vi "WriteCommand.vi"(7 "PWM":u8=24, 8 "error in":errorcluster, 9 "Com_Escribir":T1=enum."GET REF", 10 "VisaRef":refnum<vi>, 11 "Array_u8":u8[](array[numeric])) -> (0 "error out":errorcluster, 2 "VISA resource name 2":refnum<visa-resource-name>)   [LabVIEW 2026]
uses:
  Control/Ctrl_EscrituraComandos.ctl
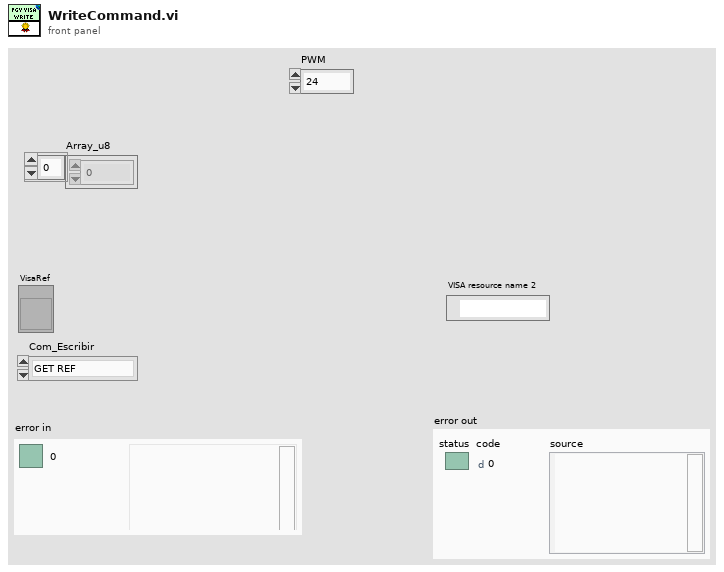
[diagram p1: front panel]
types:
  T1 = typedef "Ctrl_EscrituraComandos.ctl" = enum16{"EMERGENCY STOP", "GET REF", "SEND ROUTINE", "MOVE MANUAL", "SEND ESP32", "SET REF"}
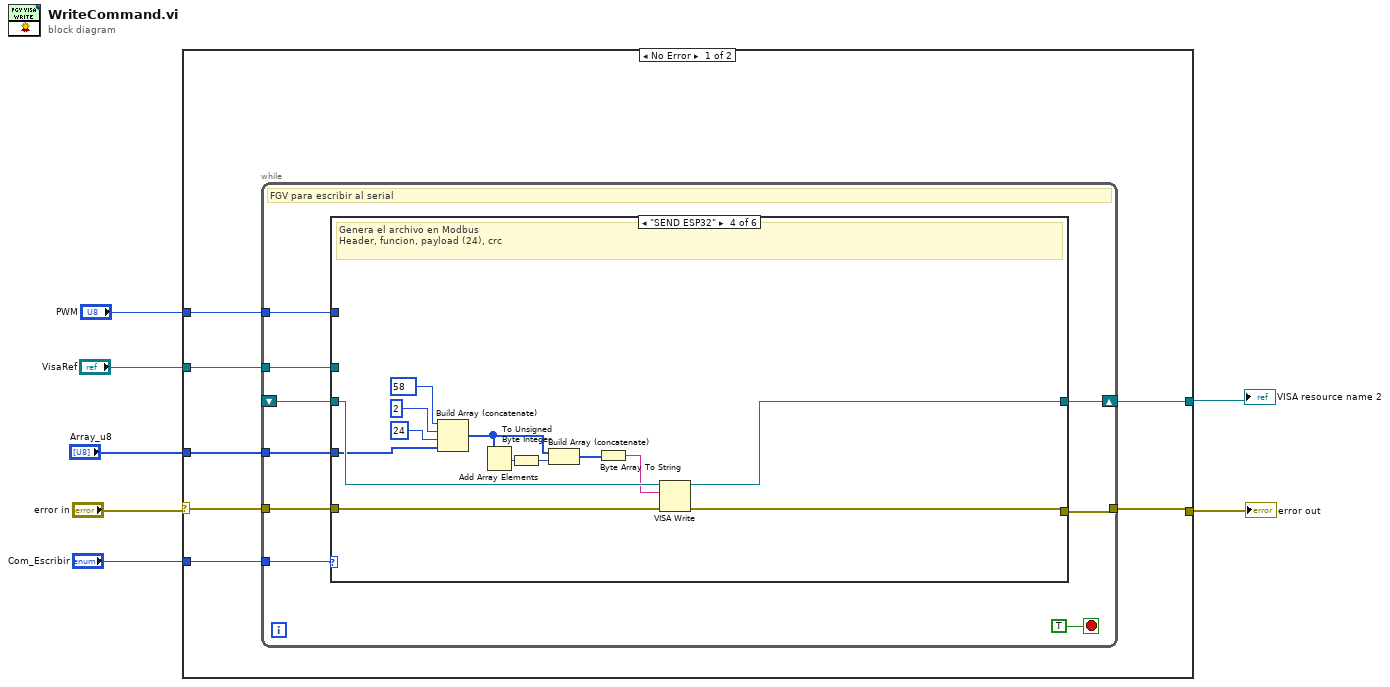
[diagram p0: block diagram]
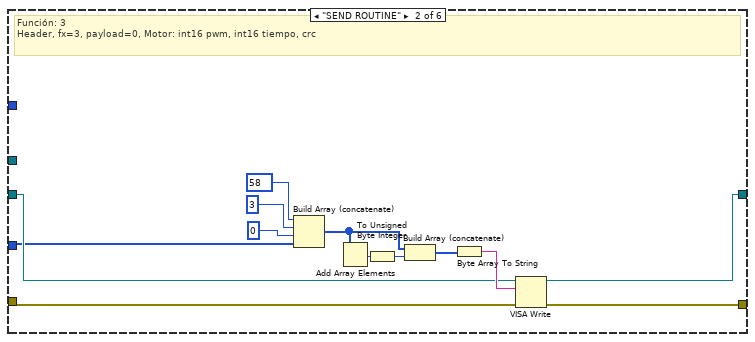
[diagram p3: hidden frame]
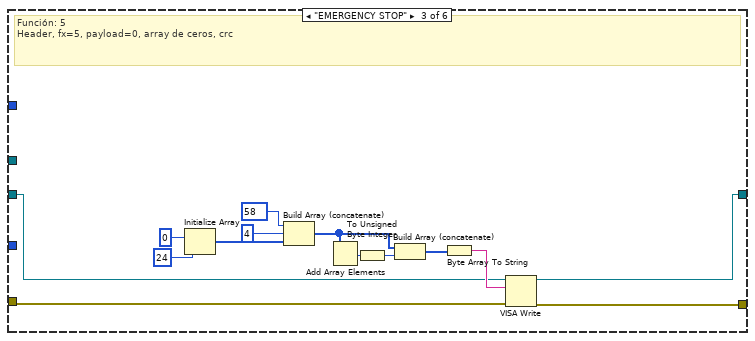
[diagram p4: hidden frame]
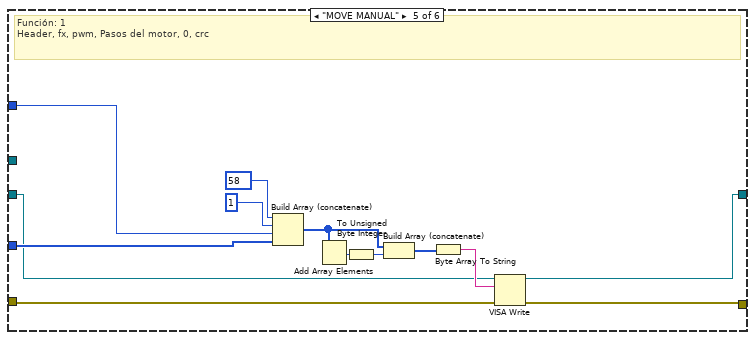
[diagram p5: hidden frame]
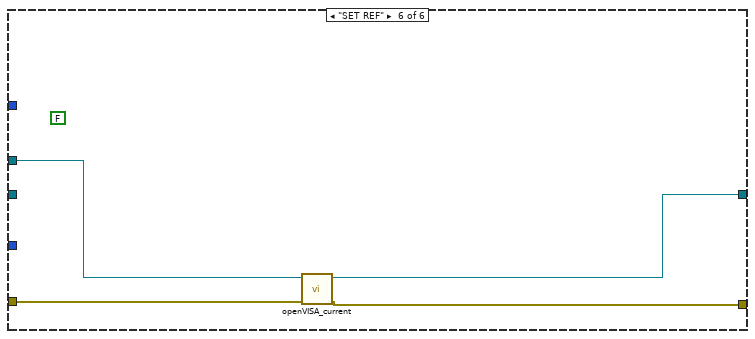
[diagram p6: hidden frame]
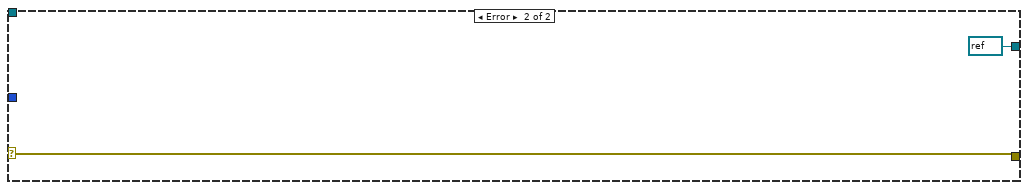
[diagram p7: hidden frame]
diagram:
  n1 = case shown="No Error" "error in" {
    selector: "error in" -> [w14 w84]
    tunnel: [w13 w84] -> w6
    tunnel: [w11 refnum<visa-resource-name> refnum ("VISA Refnum out")] -> w5
    tunnel: "Com_Escribir" -> [w12 _]
    tunnel: "Array_u8" -> [w10 _]
    tunnel: "VisaRef" -> [w9 _]
    tunnel: "PWM" -> [w8 _]
    frame No Error {
      n2 = while {
        tunnel: w12 -> [w22]
        shift-right: [w18] -> w11
        shift-left: _ -> [w19]
        tunnel: w10 -> [w20]
        tunnel: w14 -> [w21]
        tunnel: [w17] -> w13
        tunnel: w9 -> [w16]
        tunnel: w8 -> [w15]
        stop <- TRUE stop-if-true
        # "FGV para escribir al serial"
        n3 = case shown="\"SEND ESP32\"" w22 {
          tunnel: [w25 w31 w45 w64 w71 w81] -> w17
          tunnel: w21 -> [w25 w30 w42 w65 w70 w82]
          tunnel: [w24 w28 w44 w63 w67 w80] -> w18
          tunnel: w19 -> [w24 w29 w43 w62 w68 _]
          tunnel: w20 -> [_ w27 _ w58 w69 _]
          tunnel: w16 -> [_ _ _ _ _ w79]
          tunnel: w15 -> [_ _ _ _ w66 _]
          frame "GET REF" {
          }
          frame "SEND ROUTINE" {
            # "Función: 3\nHeader, fx=3, payload=0, Motor: int16 pwm, int16 tiempo, crc"
            n4 = Build Array (concatenate)(u8 58 ("element"), u8 3 ("element"), u8 0 ("element"), w27) -> (w34:u8[])
            n5 = Add Array Elements(numeric array=w34) -> (sum=w35:u8)
            n6 = To Unsigned Byte Integer(number=w35) -> (unsigned 8bit integer=w32:u8)
            n7 = Build Array (concatenate)(w34, w32) -> (w33:u8[])
            n8 = Byte Array To String(unsigned byte array=w33) -> (string=w36:string)
            n9 = VISA Write(VISA resource name=w29, write buffer=w36, error in (no error)=w30) -> (VISA resource name out=w28:refnum<visa-resource-name>, error out=w31:errorcluster)  [unwired: 1 out]
          }
          frame "EMERGENCY STOP" {
            # "Función: 5\nHeader, fx=5, payload=0, array de ceros, crc"
            n10 = Initialize Array(u8 0 ("element"), 24 ("dimension size")) -> (w39:u8[])
            n11 = Build Array (concatenate)(u8 58 ("element"), u8 4 ("element"), w39) -> (w48:u8[])
            n12 = Add Array Elements(numeric array=w48) -> (sum=w49:u8)
            n13 = To Unsigned Byte Integer(number=w49) -> (unsigned 8bit integer=w46:u8)
            n14 = Build Array (concatenate)(w48, w46) -> (w47:u8[])
            n15 = Byte Array To String(unsigned byte array=w47) -> (string=w50:string)
            n16 = VISA Write(VISA resource name=w43, write buffer=w50, error in (no error)=w42) -> (VISA resource name out=w44:refnum<visa-resource-name>, error out=w45:errorcluster)  [unwired: 1 out]
          }
          frame "SEND ESP32" {
            # "Genera el archivo en Modbus\nHeader, funcion, payload (24), crc"
            n17 = Build Array (concatenate)(u8 58 ("element"), u8 2 ("element"), u8 24 ("element"), w58) -> (w55:u8[])
            n18 = Add Array Elements(numeric array=w55) -> (sum=w56:u8)
            n19 = To Unsigned Byte Integer(number=w56) -> (unsigned 8bit integer=w53:u8)
            n20 = Build Array (concatenate)(w55, w53) -> (w54:u8[])
            n21 = Byte Array To String(unsigned byte array=w54) -> (string=w57:string)
            n22 = VISA Write(VISA resource name=w62, write buffer=w57, error in (no error)=w65) -> (VISA resource name out=w63:refnum<visa-resource-name>, error out=w64:errorcluster)  [unwired: 1 out]
          }
          frame "MOVE MANUAL" {
            # "Función: 1\nHeader, fx, pwm, Pasos del motor, 0, crc"
            n23 = Build Array (concatenate)(u8 58 ("element"), u8 1 ("element"), w66, w69) -> (w74:u8[])
            n24 = Add Array Elements(numeric array=w74) -> (sum=w75:u8)
            n25 = To Unsigned Byte Integer(number=w75) -> (unsigned 8bit integer=w72:u8)
            n26 = Build Array (concatenate)(w74, w72) -> (w73:u8[])
            n27 = Byte Array To String(unsigned byte array=w73) -> (string=w76:string)
            n28 = VISA Write(VISA resource name=w68, write buffer=w76, error in (no error)=w70) -> (VISA resource name out=w67:refnum<visa-resource-name>, error out=w71:errorcluster)  [unwired: 1 out]
          }
          frame "SET REF" {
            (unwired) FALSE
            n29 = call "openVISA_current.vi"("error in (no error)"=w82, "VisaRef"=w79) -> ("error out"=w81:errorcluster, "VISA Refnum out"=w80:refnum<visa-resource-name>)  [unwired: 8 in]
          }
        }
      }
    }
    frame Error {
    }
  }
  "error out" <- w6
  "VISA resource name 2" <- w5
